vi "Smooth Background DBL.vi"(7 "Type":T1(ring)=enum."Bandpass", 8 "Error In":errorcluster, 9 "HP F":dbl format="%#_6p", 10 "LP  F":dbl=0.001 format="%#_6p", 11 "Data":dbl[](array[numeric])) -> (0 "Error Out":errorcluster, 3 "Data out":dbl[](array[numeric]))   [LabVIEW 2016]
uses:
  <vilib>/measure/NI_MAPro.lvlib
  <vilib>/Analysis/3filter.llb/Filter Structure Type.ctl
  <vilib>/Analysis/NI_AALBase.lvlib
  <vilib>/measure/macond.llb/IIR Filter for 1 Chan.vi
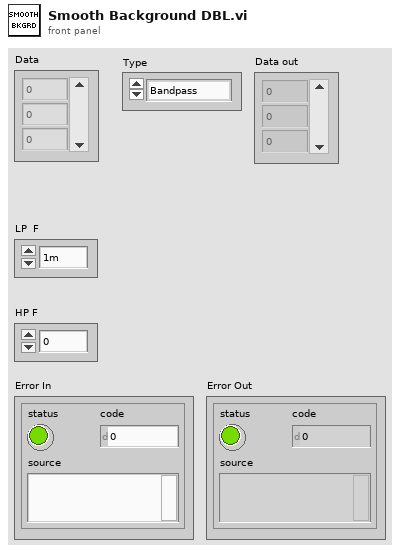
[diagram p1: front panel]
types:
  T1 = enum16{"Lowpass", "Highpass", "Bandpass", "Bandstop"}
  T2 = typedef "NI_AALBase.lvlib/Filter Structure Type.ctl" = u16
  T3 = cluster{"Topology":enum16{"Off", "Butterworth", "Chebyshev", "Inverse Chebyshev", "Elliptic", "Bessel"}, "Type":enum16{"Lowpass", "Highpass", "Bandpass", "Bandstop"}, "Order":i32, "Lower Fc":dbl, "Upper Fc":dbl, "PB Ripple":dbl, "SB Attenuation":dbl}
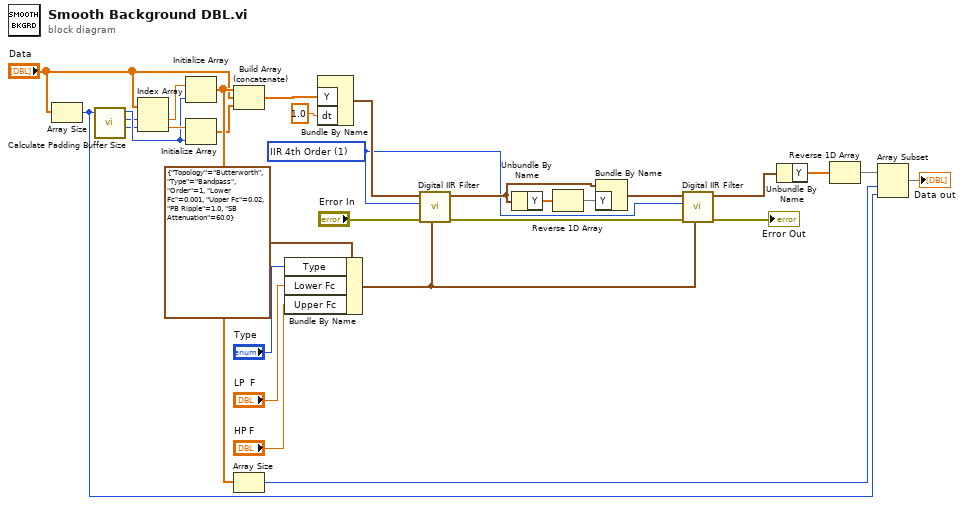
[diagram p0: block diagram]
diagram:
  w17 = T2 1 items=["IIR 2nd Order"=0, "IIR 4th Order"=1, "Auto Select"=10] ("filter structure option")
  n1 = Array Size(array="Data") -> (size(s)=w4:i32)
  n2 = call "Calculate Padding Buffer Size.vi"("Array size"=w4) -> ("Last element"=w1:i32, "First element"=w2:i32, "Buffer size"=w3:i32)  [unwired: 8 in]
  n3 = Index Array(array="Data", index #1=w2, index #2=w1) -> (element #1=w28:dbl, element #2=w9:dbl)
  n4 = Initialize Array(w28, w3) -> (w30:dbl[])
  n5 = Initialize Array(w9, w3) -> (w8:dbl[])
  n6 = Build Array (concatenate)(w30, "Data", w8) -> (w29:dbl[])
  n7 = Array Size(array=w30) -> (size(s)=w12:i32)
  n8 = Bundle By Name(cluster=T3 {"Topology"=enum."Butterworth", "Type"=enum."Bandpass", "Order"=1, "Lower Fc"=0.001, "Upper Fc"=0.02, "PB Ripple"=1.0, "SB Attenuation"=60.0} ("IIR filter specifications"), "Type"="Type", "Lower Fc"="LP  F", "Upper Fc"="HP F") -> (w18:T3)
  n9 = Bundle By Name("Y"=w29, "dt"=1.0) -> (w26:waveform(dbl))  [unwired: 1 in]
  n10 = call-poly <vilib>:"Digital IIR Filter.vi"("IIR filter specifications"=w18, "error in (no error)"="Error In", "filter structure option"=w17, "signal in"=w26) -> ("error out"=w16:errorcluster, "signal out"=w21:waveform(dbl))  [unwired: 5 in, 1 out]
  n11 = Unbundle By Name(w21) -> ("Y"=w22:dbl[])
  n12 = Reverse 1D Array(array=w22) -> (reversed array=w20:dbl[])
  n13 = Bundle By Name(cluster=w21, "Y"=w20) -> (w19:waveform(dbl))
  n14 = call-poly <vilib>:"Digital IIR Filter.vi"("IIR filter specifications"=w18, "error in (no error)"=w16, "filter structure option"=w17, "signal in"=w19) -> ("error out"=→"Error Out":errorcluster, "signal out"=w14:waveform(dbl))  [unwired: 5 in, 1 out]
  n15 = Unbundle By Name(w14) -> ("Y"=w15:dbl[])
  n16 = Reverse 1D Array(array=w15) -> (reversed array=w13:dbl[])
  n17 = Array Subset(array=w13, index=w12, length=w4) -> (→"Data out":dbl[])
